vi "solar Target by Name.vi"(7 "Default LVClass":refnum<class "solar.lvclass">, 8 "error in (no error)":errorcluster, 10 "LVClass (*.lvclass)":string, 11 "Target Name":string) -> (0 "error out":errorcluster, 3 "solar":refnum<class "solar.lvclass">)   [LabVIEW 2018]
doc: "This loads a Target by LabVIEW Class and Target Name name. This is useful for loading the Target's LVClass in another target. The solar private class data is contained in a single element queue so all data is referenced by pointers allowing the target to be loaded by name."
uses:
  solar.lvclass
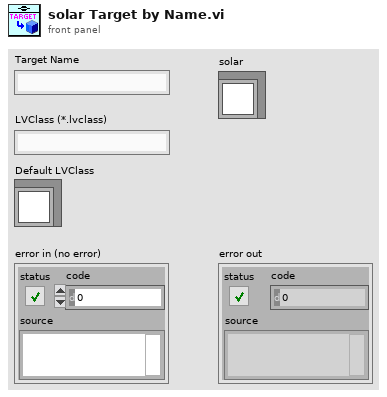
[diagram p1: front panel]
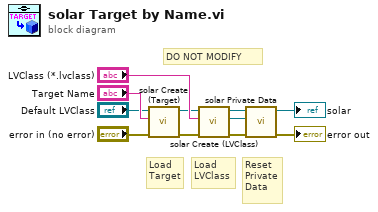
[diagram p0: block diagram]
diagram:
  # "Reset\nPrivate\nData"
  # "DO NOT MODIFY"
  # "Load\nLVClass"
  # "Load\nTarget"
  n1 = call "solar Create (Target).vi"("error in (no error)"="error in (no error)", "Target Name"="Target Name", "Default LVClass"="Default LVClass") -> ("error out"=w8:errorcluster, "solar"=w7:refnum<class "solar.lvclass">)  [unwired: 7 in]
  n2 = call "solar Create (LVClass).vi"("error in (no error)"=w8, "LVClass (*.lvclass)"="LVClass (*.lvclass)", "Default LVClass"=w7) -> ("error out"=w5:errorcluster, "dup Default LVClass"=w2:refnum<class "solar.lvclass">, "solar out"=w4:refnum<class "solar.lvclass">)  [unwired: 6 in]
  n3 = call-dynamic "solar Private Data.vi"("error in (no error)"=w5, "Default LVClass"=w2, "solar in"=w4) -> ("error out"=→"error out":errorcluster, "solar out"=→"solar":refnum<class "solar.lvclass">)  [unwired: 7 in]
